vi "main.vi"() -> ()   [LabVIEW 2023]
uses:
  CONTROLS/states.ctl
panel:
  out "Meldung":string
  out "Enum":T1
  in  "stop":bool
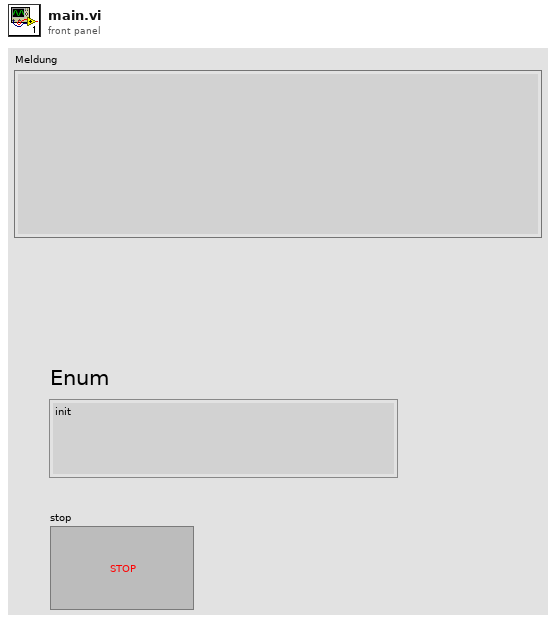
[diagram p1: front panel]
types:
  T1 = typedef "states.ctl" = enum16{"init", "read", "write", "Kundeneingabe", "Betonauswahl", "Bezahlprozeß", "Rechnung", "Zudaten mit Gewichtmessung", "Stop"}
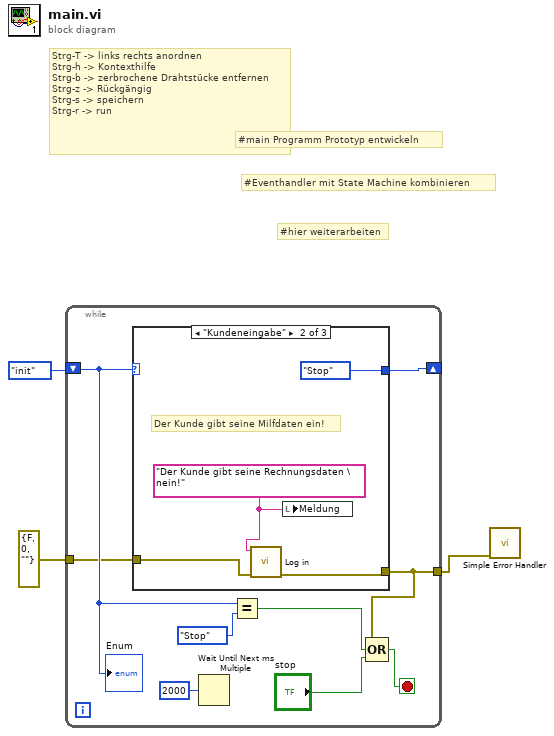
[diagram p0: block diagram]
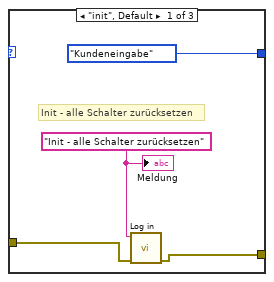
[diagram p2: hidden frame]
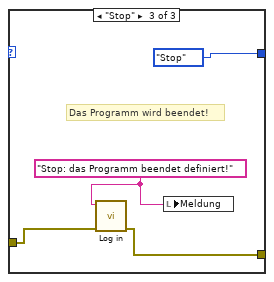
[diagram p3: hidden frame]
diagram:
  # "#hier weiterarbeiten"
  # "#Eventhandler mit State Machine kombinieren"
  # "#main Programm Prototyp entwickeln"
  # "Strg-T -> links rechts anordnen\nStrg-h -> Kontexthilfe\nStrg-b -> zerbrochene Drahtstücke entfernen\nStrg-z -> Rückgängig\nStrg-s -> speichern\nStrg-r -> run"
  n1 = while {
    shift-right: [w12] -> _
    shift-left: states."init" -> [w10]
    tunnel: errorcluster {"status"=FALSE, "code"=0, "source"=""} ("error in") -> [w5]
    tunnel: [w4] -> w1
    stop <- w7 stop-if-true
    n2 = case shown="\"Kundeneingabe\"" w10 {
      tunnel: [states."Kundeneingabe" states."Stop" states."Stop"] -> w12
      tunnel: w5 -> [w14 w18 w22]
      tunnel: [w13 w17 w21] -> w4
      frame "init", Default {
        w15 = "Init - alle Schalter zurücksetzen" ("Meldung")
        # "Init - alle Schalter zurücksetzen"
        n3 = call "Log in.vi"("error in"=w14, "log"=w15) -> ("error out"=w13:errorcluster)  [unwired: 9 in]
        "Meldung" <- w15
      }
      frame "Kundeneingabe" {
        w19 = "Der Kunde gibt seine Rechnungsdaten \nein!" ("Meldung")
        # "Der Kunde gibt seine Milfdaten ein!"
        n4 = call "Log in.vi"("error in"=w18, "log"=w19) -> ("error out"=w17:errorcluster)  [unwired: 9 in]
        n5 = local write "Meldung"(w19) -> ()
      }
      frame "Stop" {
        w23 = "Stop: das Programm beendet definiert!" ("Meldung")
        # "Das Programm wird beendet!"
        n6 = call "Log in.vi"("error in"=w22, "log"=w23) -> ("error out"=w21:errorcluster)  [unwired: 9 in]
        n7 = local write "Meldung"(w23) -> ()
      }
    }
    n8 = Wait Until Next ms Multiple(millisecond multiple=u32 2000) -> ()  [unwired: 1 out]
    n9 = Equal?(x=w10, y=states."Stop") -> (x = y?=w9:bool)
    n10 = Compound Arithmetic op=OR(w4, w9, "stop") -> (w7:bool)
    "Enum" <- w10
  }
  n11 = call <vilib>:"Simple Error Handler.vi"("error in (no error)"=w1) -> ()  [unwired: 4 in, 5 out]
